vi "hmi_shutdown.vi"(7 "hmi_references":T1, 8 "error in (no error)":errorcluster) -> (0 "error out":errorcluster)   [LabVIEW 2015, in "lv-interface-re.lvlib"]
uses:
  lv-interface-re.lvlib
  _controls/hmi_references.ctl
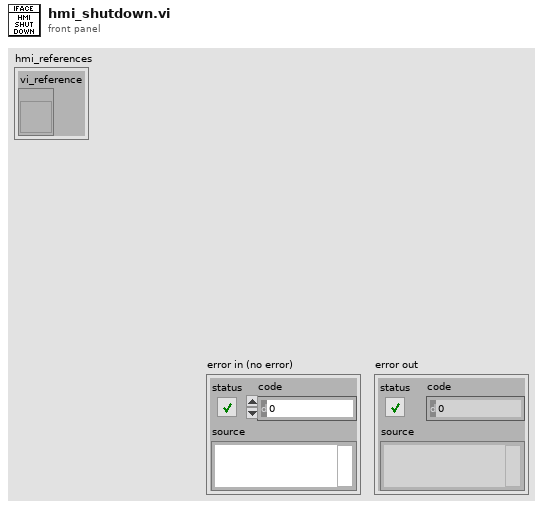
[diagram p1: front panel]
types:
  T1 = typedef "lv-interface-re.lvlib/hmi_references.ctl" = cluster{"vi_reference":refnum<vi>}
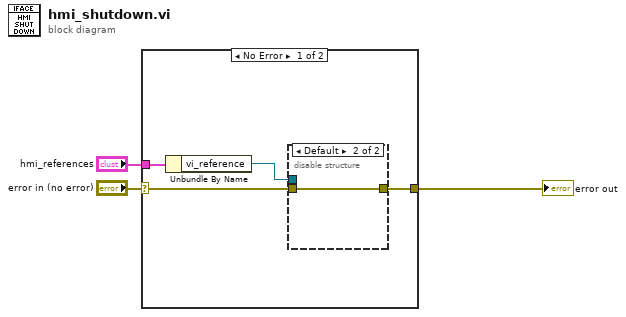
[diagram p0: block diagram]
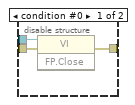
[diagram p2: hidden frame]
diagram:
  n1 = case shown="No Error" "error in (no error)" {
    selector: "error in (no error)" -> [w4 w12]
    tunnel: [w6 w12] -> w2
    tunnel: "hmi_references" -> [w5 _]
    frame No Error {
      n2 = Unbundle By Name(w5) -> ("vi_reference"=w7:refnum<vi>)
      n3 = disable-structure shown="Default" {
        disable-tunnel: w7 -> [w10 _]
        disable-tunnel: w4 -> [w9 w11]
        disable-tunnel: [w8 w11] -> w6
        frame condition #0 {
          n4 = invoke class="VI" method="FP.Close"(reference=w10, error in=w9) -> (error out=w8:errorcluster)  [unwired: 1 in, 2 out]
        }
        frame condition #1 (active) {
        }
      }
    }
    frame Error {
    }
  }
  "error out" <- w2
